vi "createActuator.vi"(8 "error in (no error)":errorcluster, 11 "Controller in":refnum<class "Controller.lvclass">) -> (0 "error out":errorcluster, 2 "Actuator":refnum<class "IActuator.lvclass">, 3 "Controller out":refnum<class "Controller.lvclass">)   [LabVIEW 2015, in "Controller.lvclass"]
uses:
  Controller.lvclass
  Model/Actuator/IActuator/IActuator.lvclass
  Model/ActuatorCylinder/PressureServoActuatorCylinder/PressureServoCylinderActuator.lvclass
  Model/ActuatorCylinder/ILCControlledActuatorCylinder/ILCControlledActuatorCylinder.lvclass
  Model/ILCDACFactory/ILCDACFactory/ILCDACFactory.lvclass
  Model/ActuatorCylinder/PressureServoActuatorCylinder/PressureServoCylinderActuator.lvclass/PressureServoCylinderActuator.ctl
  Model/ActuatorCylinder/ILCControlledActuatorCylinder/ILCControlledActuatorCylinder.lvclass/ILCControlledActuatorCylinder.ctl
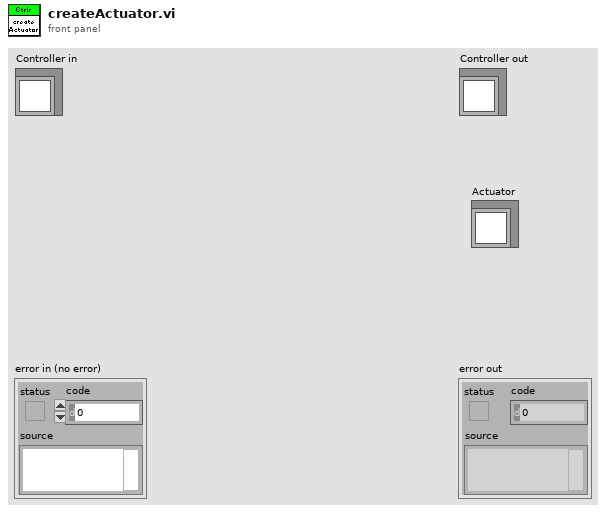
[diagram p1: front panel]
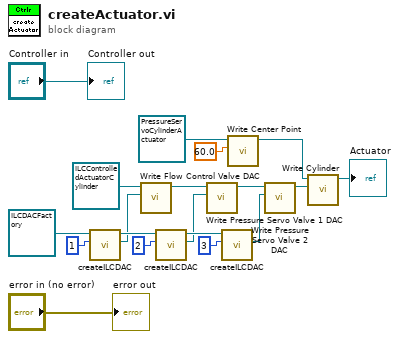
[diagram p0: block diagram]
diagram:
  n1 = call-dynamic "createILCDAC.vi"("Channel"=u8 1, "ILCDACFactory in"=refnum<class "ILCDACFactory.lvclass"> refnum ("ILCDACFactory.lvclass")) -> ("ILCDAC"=w6:refnum<class "IILCDAC.lvclass">, "ILCDACFactory out"=w8:refnum<class "ILCDACFactory.lvclass">)  [unwired: 7 in, 1 out]
  n2 = call "Write Flow Control Valve DAC.vi"("IILCDAC"=w6, "ILCControlledActuatorCylinder in"=refnum<class "ILCControlledActuatorCylinder.lvclass"> refnum ("ILCControlledActuatorCylinder.lvclass")) -> ("ILCControlledActuatorCylinder out"=w12:refnum<class "ILCControlledActuatorCylinder.lvclass">)  [unwired: 9 in]
  n3 = call-dynamic "createILCDAC.vi"("Channel"=u8 2, "ILCDACFactory in"=w8) -> ("ILCDAC"=w5:refnum<class "IILCDAC.lvclass">, "ILCDACFactory out"=w7:refnum<class "ILCDACFactory.lvclass">)  [unwired: 7 in, 1 out]
  n4 = call "Write Pressure Servo Valve 1 DAC.vi"("IILCDAC"=w5, "ILCControlledActuatorCylinder in"=w12) -> ("ILCControlledActuatorCylinder out"=w13:refnum<class "ILCControlledActuatorCylinder.lvclass">)  [unwired: 9 in]
  n5 = call-dynamic "createILCDAC.vi"("Channel"=u8 3, "ILCDACFactory in"=w7) -> ("ILCDAC"=w4:refnum<class "IILCDAC.lvclass">)  [unwired: 7 in, 2 out]
  n6 = call "Write Center Point.vi"("Center Point"=dbl[unit] 60.0, "PressureServoCylinderActuator in"=refnum<class "PressureServoCylinderActuator.lvclass"> refnum ("PressureServoCylinderActuator.lvclass")) -> ("PressureServoCylinderActuator out"=w15:refnum<class "PressureServoCylinderActuator.lvclass">)  [unwired: 9 in]
  n7 = call "Write Pressure Servo Valve 2 DAC.vi"("IILCDAC"=w4, "ILCControlledActuatorCylinder in"=w13) -> ("ILCControlledActuatorCylinder out"=w10:refnum<class "ILCControlledActuatorCylinder.lvclass">)  [unwired: 9 in]
  n8 = call "Write Cylinder.vi"("IActuatorCylinder.lvclass"=w10, "PressureServoCylinderActuator in"=w15) -> ("PressureServoCylinderActuator out"=→"Actuator":refnum<class "PressureServoCylinderActuator.lvclass">)  [unwired: 9 in]
  "error out" <- "error in (no error)"
  "Controller out" <- "Controller in"
